vi "GlobalGetTimingsFromCamera.vi"() -> ()   [LabVIEW 2011]
panel:
  in  "Accumulation Camera 1":dbl
  in  "Kinetics Camera 1":dbl
  in  "Exposure Camera 1":dbl
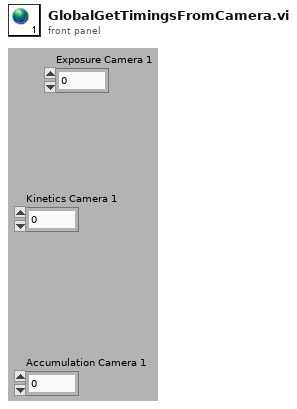
[diagram p1: front panel]
diagram:
